vi "ChildModule.Exit.vi"(8 "error in":errorcluster) -> (0 "error out":errorcluster)   [LabVIEW 2016]
uses:
  <vilib>/KATE/Queues/Queue Utils.lvlib
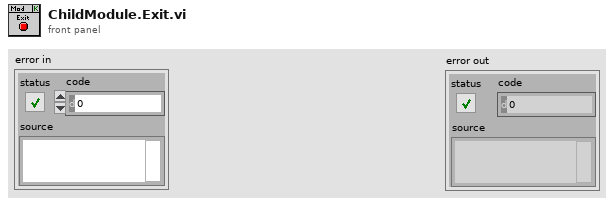
[diagram p1: front panel]
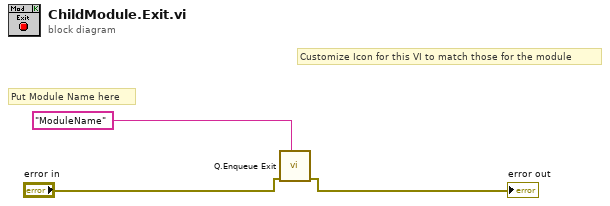
[diagram p0: block diagram]
diagram:
  # "Customize Icon for this VI to match those for the module"
  # "Put Module Name here"
  n1 = call <vilib>:"Q.Enqueue Exit.vi"("Q Name"="ModuleName", "Error In"="error in") -> ("error out"=→"error out":errorcluster)  [unwired: 8 in, 1 out]
